vi "Create Function String.vi"   [LabVIEW 2021, in "Yokogawa WT1800 Series.lvlib"]
doc: "Create a Function string used as an input <b>Function</b> in the <b>Configure Numeric (Normal) VI</b> and <b>Configure User Defined Event (Range) VI</b>"
uses:
  <instrlib>/Yokogawa WT1800 Series/Yokogawa WT1800 Series.lvlib
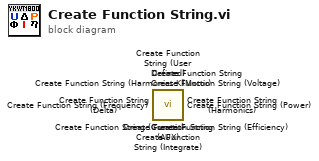
[diagram p0: block diagram]
diagram:
  n1 = call <instrlib>:"Create Function String (AUX).vi"() -> ()  [unwired: 9 in, 3 out]
  n2 = call <instrlib>:"Create Function String (Motor).vi"() -> ()  [unwired: 9 in, 3 out]
  n3 = call <instrlib>:"Create Function String (Delta).vi"() -> ()  [unwired: 9 in, 3 out]
  n4 = call <instrlib>:"Create Function String (Harmonics).vi"() -> ()  [unwired: 9 in, 3 out]
  n5 = call <instrlib>:"Create Function String (Harmonics K).vi"() -> ()  [unwired: 9 in, 3 out]
  n6 = call <instrlib>:"Create Function String (User Defined).vi"() -> ()  [unwired: 9 in, 3 out]
  n7 = call <instrlib>:"Create Function String (Efficiency).vi"() -> ()  [unwired: 9 in, 3 out]
  n8 = call <instrlib>:"Create Function String (Integrate).vi"() -> ()  [unwired: 9 in, 3 out]
  n9 = call <instrlib>:"Create Function String (Frequency).vi"() -> ()  [unwired: 9 in, 3 out]
  n10 = call <instrlib>:"Create Function String (Power).vi"() -> ()  [unwired: 9 in, 3 out]
  n11 = call <instrlib>:"Create Function String (Current).vi"() -> ()  [unwired: 9 in, 3 out]
  n12 = call <instrlib>:"Create Function String (Voltage).vi"() -> ()  [unwired: 9 in, 3 out]
